vi "Rect32ToBounds.vi"(1 "Rect32":T3) -> (0 "Bounds":T1)   [LabVIEW 2020, in "NI_XNodeSupport.lvlib"]
uses:
  NI_XNodeSupport.lvlib
  XNodeRect32.ctl
  XNodeInt.ctl
  XNodeBounds.ctl
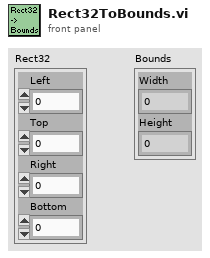
[diagram p1: front panel]
types:
  T1 = typedef "NI_XNodeSupport.lvlib/XNodeBounds.ctl" = cluster{"Width":T2, "Height":T2}
  T2 = typedef "NI_XNodeSupport.lvlib/XNodeInt.ctl" = i32
  T3 = typedef "NI_XNodeSupport.lvlib/XNodeRect32.ctl" = cluster{"Left":T2, "Top":T2, "Right":T2, "Bottom":T2}
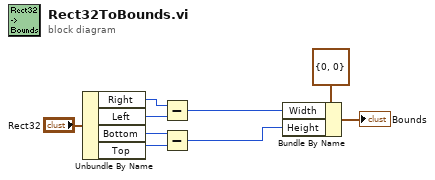
[diagram p0: block diagram]
diagram:
  n1 = Unbundle By Name("Rect32") -> ("Right"=w7:T2, "Left"=w6:T2, "Bottom"=w5:T2, "Top"=w4:T2)
  n2 = Subtract(x=w7, y=w6) -> (x-y=w2:T2)
  n3 = Subtract(x=w5, y=w4) -> (x-y=w3:T2)
  n4 = Bundle By Name(cluster=T1 {"Width"=0, "Height"=0} ("Bounds"), "Width"=w2, "Height"=w3) -> (→"Bounds":T1)
